vi "Center Spin.vi"(0 "RobotDriveDevRef":T1={"DevStatus"={"status"=FALSE, "code"=0, "source"=""}, "Motors[]"=[], "Square Inputs"=FALSE, "Max Output"=1.0, "Isochronous"=FALSE}, 1 "RobotPivotDevRef":T1={"DevStatus"={"status"=FALSE, "code"=0, "source"=""}, "Motors[]"=[], "Square Inputs"=FALSE, "Max Output"=1.0, "Isochronous"=FALSE}, 2 "Width":dbl, 3 "Legnth":dbl, 4 "Joystick axis":dbl, 5 "error in (no error)":errorcluster, 7 "Rear Left Current Pivot Angle":dbl, 9 "Rear Right Current Pivot Angle":dbl, 11 "Front Left Current Pivot Angle":dbl, 13 "Front Right Current Pivot Angle":dbl) -> (14 "RobotPivotDevRef Out":T1={"DevStatus"={"status"=FALSE, "code"=0, "source"=""}, "Motors[]"=[], "Square Inputs"=FALSE, "Max Output"=1.0, "Isochronous"=FALSE}, 15 "RobotDriveDevRef Out":T1={"DevStatus"={"status"=FALSE, "code"=0, "source"=""}, "Motors[]"=[], "Square Inputs"=FALSE, "Max Output"=1.0, "Isochronous"=FALSE}, 19 "error out":errorcluster)   [LabVIEW 2011, in "Pivot Drive.lvlib"]
doc: "A convience VI. This will make the robot spin around it's center. This implements the pivot drive VI, in a way so not as many inputs or calculations are required."
uses:
  Pivot Drive.lvlib
  <vilib>/Rock Robotics/WPI/RobotDrive/WPI_RobotDriveDevRef.ctl
  <vilib>/Rock Robotics/WPI/MotorControl/WPI_MotorControlDeviceRef.ctl
  <vilib>/Rock Robotics/SystemInterfaces/Typedef/FPGA_TypedefDigitalModule.ctl
  <vilib>/Rock Robotics/SystemInterfaces/DIO/FPGA_DIOPWMChannel.ctl
  <vilib>/Rock Robotics/WPI/PWM/WPI_PWMDeadband.ctl
  <vilib>/Rock Robotics/WPI/CAN/Jaguar/SubVIs/WPI_CANJaguar_ControlMode.ctl
  <vilib>/Rock Robotics/WPI/PWM/WPI_PWMTransform_ConPane.ctl
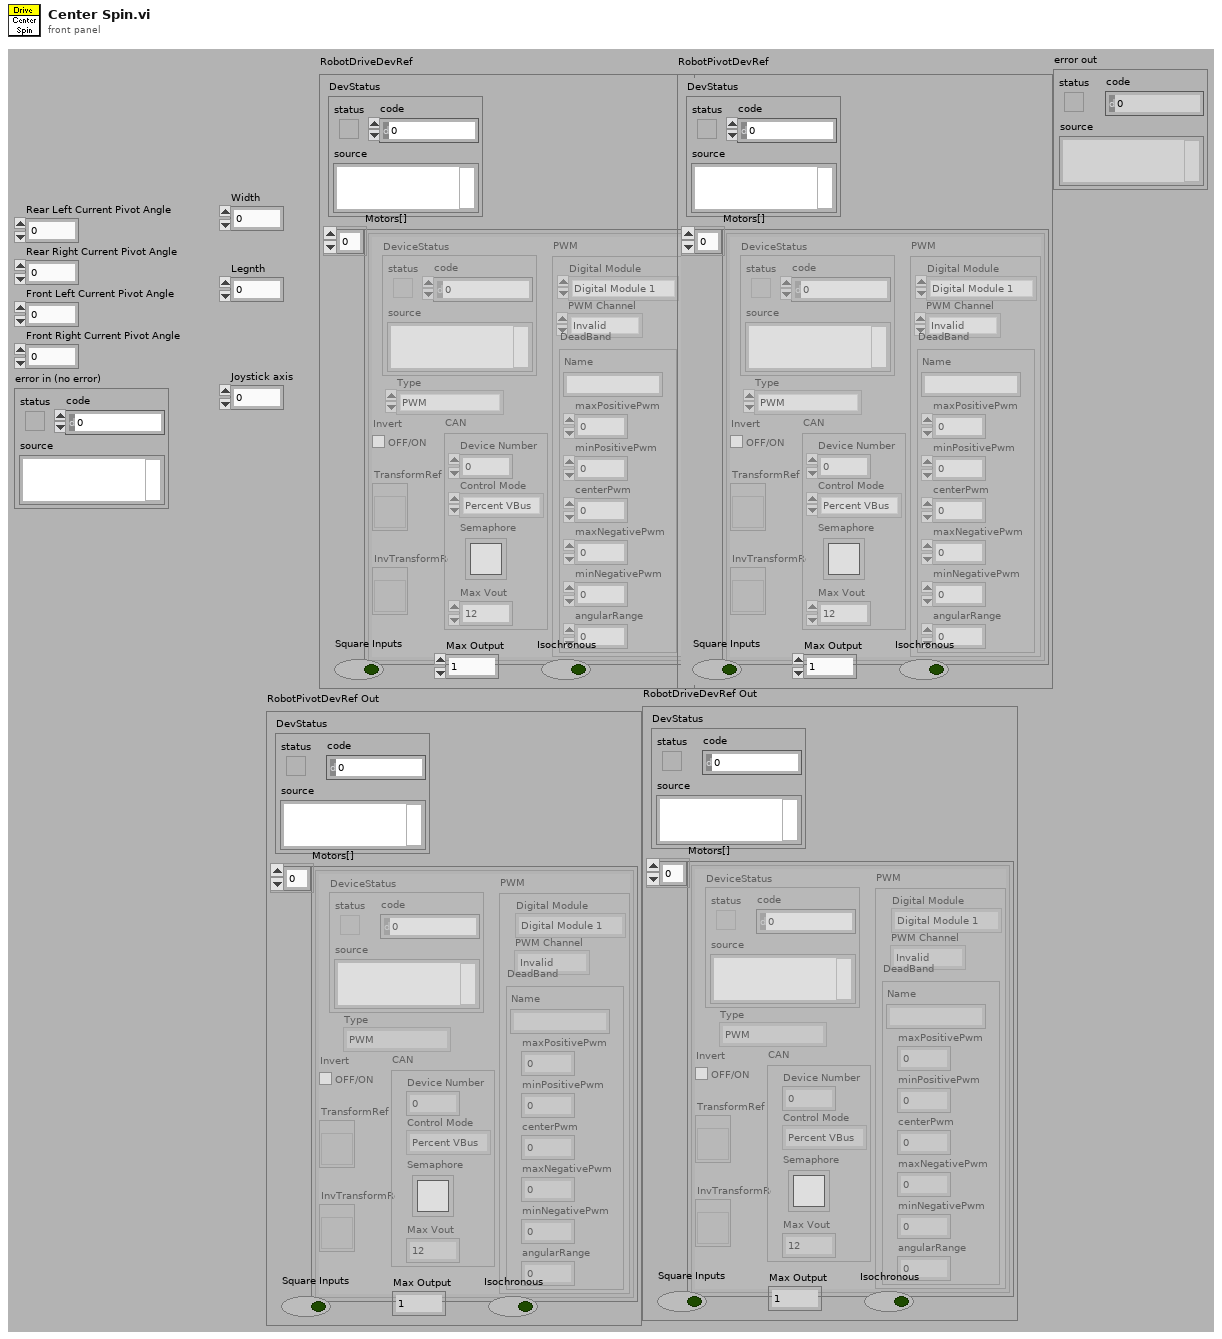
[diagram p1: front panel]
types:
  T1 = typedef "WPI_RobotDriveDevRef.ctl" = cluster{"DevStatus":errorcluster, "Motors[]":T2[], "Square Inputs":bool, "Max Output":dbl, "Isochronous":bool}
  T2 = typedef "WPI_MotorControlDeviceRef.ctl" = cluster{"DeviceStatus":errorcluster, "Type":enum16{"PWM", "CAN"}, "PWM":cluster{"Digital Module":T3, "PWM Channel":T4, "DeadBand":T5}, "CAN":cluster{"Device Number":u8, "Control Mode":T6, "Semaphore":T7, "Max Vout":dbl}, "Invert":bool, "TransformRef":T8, "InvTransformRef":T8}
  T3 = typedef "FPGA_TypedefDigitalModule.ctl" = enum16{"Digital Module 1", "Digital Module 2"}
  T4 = typedef "FPGA_DIOPWMChannel.ctl" = enum8{"PWM 1", "PWM 2", "PWM 3", "PWM 4", "PWM 5", "PWM 6", "PWM 7", "PWM 8", "PWM 9", "PWM 10", "Invalid"}
  T5 = typedef "WPI_PWMDeadband.ctl" = cluster{"Name":string, "maxPositivePwm":i32, "minPositivePwm":i32, "centerPwm":i32, "maxNegativePwm":i32, "minNegativePwm":i32, "angularRange":u16}
  T6 = typedef "WPI_CANJaguar_ControlMode.ctl" = enum8{"Percent VBus", "Current", "Speed", "Position", "Voltage"}
  T7 = typedef "Semaphore RefNum" = refnum<k1>
  T8 = typedef "WPI_PWMTransform_ConPane.ctl" = refnum<vi>
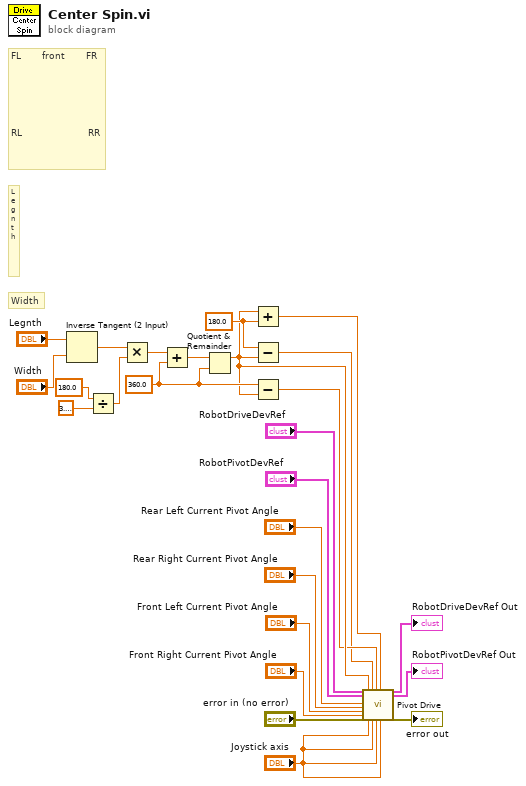
[diagram p0: block diagram]
diagram:
  w7 = 180.0
  w5 = 360.0
  # "Legnth"
  # "Width"
  # "FL       front       FR\n\n\n\n\n\n\nRL                      RR"
  n1 = Inverse Tangent (2 Input)(1:"Width", 2:"Legnth") -> (0:w20:dbl)
  n2 = Divide(x=180.0, y=3.141592653589793) -> (x/y=w21:dbl)
  n3 = Multiply(x=w20, y=w21) -> (x*y=w8:dbl)
  n4 = Add(x=w8, y=w5) -> (x+y=w6:dbl)
  n5 = Quotient & Remainder(x=w6, y=w5) -> (x-y*floor(x/y)=w4:dbl)  [unwired: 1 out]
  n6 = Add(x=w4, y=w7) -> (x+y=w3:dbl)
  n7 = Subtract(x=w7, y=w4) -> (x-y=w1:dbl)
  n8 = Subtract(x=w5, y=w4) -> (x-y=w2:dbl)
  n9 = call "Pivot Drive.vi"("RobotDriveDevRef"="RobotDriveDevRef", "RobotPivotDevRef"="RobotPivotDevRef", "Rear Left Current Pivot Angle"="Rear Left Current Pivot Angle", "Rear Right Current Pivot Angle"="Rear Right Current Pivot Angle", "Front Left Current Pivot Angle"="Front Left Current Pivot Angle", "Front Right Current Pivot Angle"="Front Right Current Pivot Angle", "error in (no error)"="error in (no error)", "Rear Left Wanted Pivot Angle"=w4, "Rear Left Speed"="Joystick axis", "Rear Right Wanted Pivot Angle"=w1, "Rear Right Speed"="Joystick axis", "Front Left Wanted Pivot Angle"=w2, "Front Left Speed"="Joystick axis", "Front Right Wanted Pivot Angle"=w3, "Front Right Speed"="Joystick axis") -> ("RobotDriveDevRef Out"=→"RobotDriveDevRef Out":T1, "RobotPivotDevRef Out"=→"RobotPivotDevRef Out":T1, "error out"=→"error out":errorcluster)  [unwired: 2 in, 8 out]
